vi "Main.vi"(8 "error in":errorcluster, 11 "ArduinoOperator in":refnum<class "ArduinoOperator.lvclass">) -> (0 "error out":errorcluster, 3 "ArduinoOperator out":refnum<class "ArduinoOperator.lvclass">)   [LabVIEW 2022 SP3, in "ArduinoOperator.lvclass"]
doc: "The Queued Message Handler of a Worker."
uses:
  ArduinoOperator.lvclass
  C:/Program Files (x86)/National Instruments/LabVIEW 2022/vi.lib/addons/_Workers/Library/Classes/Worker/Worker.lvclass
  <vilib>/addons/_Workers/Library/Classes/Worker/Worker.lvclass/Worker.ctl
  <vilib>/addons/_Workers/Library/Classes/Message/Priority.ctl
  ArduinoOperator.lvclass/ArduinoOperator.ctl
  <vilib>/MakerHub/LINX/Public/Peripherals/Analog/Analog Read 1 Chan.vi
  <vilib>/MakerHub/LINX/Public/Peripherals/Digital/Digital Read 1 Chan.vi
  <vilib>/MakerHub/LINX/Public/Peripherals/Digital/Digital Write 1 Chan.vi
  <vilib>/MakerHub/LINX/Public/Peripherals/Analog/Analog Read N Chans.vi
  <vilib>/MakerHub/LINX/Public/Peripherals/Digital/Digital Read N Chans.vi
  <vilib>/MakerHub/LINX/Public/Peripherals/Digital/Digital Write N Chans.vi
  <vilib>/MakerHub/LINX/Private/Local IO/LinxAnalogRead.vi
  <vilib>/MakerHub/LINX/Public/Utilities/Check Channel.vi
  <vilib>/MakerHub/LINX/Private/Local IO/LinxDigitalRead.vi
  <vilib>/MakerHub/LINX/Private/Local IO/LinxDigitalWrite.vi
  <vilib>/addons/_Workers/Library/Classes/Message/Enqueue Message to Self v2.vi
  <vilib>/MakerHub/LINX/Public/Utilities/Open Serial.vi
  <vilib>/MakerHub/LINX/Private/Utilties/Generate Error.vi
  <vilib>/addons/_Workers/Library/Classes/Message/Enqueue Message to Self v2 - Array.vi
  Initialization Data.ctl
  <vilib>/addons/_Workers/Library/Classes/Worker/Worker.lvclass
  <vilib>/addons/_Workers/Library/Classes/Message/Message.lvclass
  <vilib>/MakerHub/LINX/LMH-LINX.lvlib
  C:/Program Files (x86)/National Instruments/LabVIEW 2022/vi.lib/addons/_Workers/Library/Classes/Workers Object/Workers Object.lvclass
  C:/Users/chrismadlax/Desktop/LVSampleCode/ArduinoController/Workers/ArduinoOperator/ArduinoOperator.lvclass
  <vilib>/addons/_Workers/Library/Classes/Message Queue/Message Queue.lvclass
panel:
  out "Target":bool
  in  "TimerON":bool
  in  "TimerCount(ms)":i32=1000
  out "Loop Rate (Hz)":u32
  in  "Close":bool
  in  "Link":bool
  in  "AI Channel":u8
  out "Analog Data":dbl(graph)
  in  "DI Channel":u8=2
  out "DI Value":bool
  in  "DO Value":bool
  in  "DO Channel":u8=3
  in  "Serial Port":refnum<visa-resource-name>
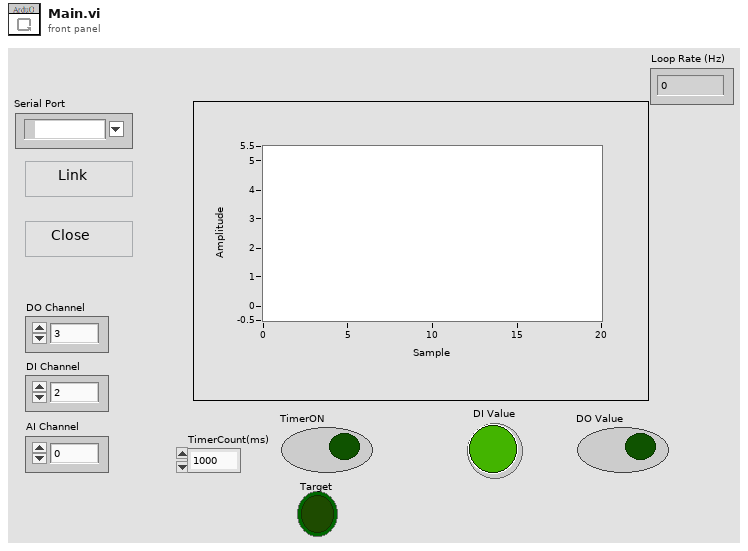
[diagram p1: front panel]
types:
  T1 = typedef "ArduinoOperator.lvclass/Initialization Data.ctl" = cluster{"String":string}
  T2 = typedef "Workers.lvlib/Message.lvclass/Priority.ctl" = enum16{"Low", "Normal", "High"}
  T3 = typedef "Workers.lvlib/Case Label.ctl" = string
  T4 = typedef "LMH-LINX.lvlib/LINX Ref.ctl" = cluster{"IO":T5, "Interface":T6, "LINX Device Config":T7}
  T5 = typedef "LMH-LINX.lvlib/Platform.ctl" = enum16{"Remote", "Local"}
  T6 = typedef "LMH-LINX.lvlib/Interface.ctl" = enum16{"Serial", "TCP"}
  T7 = typedef "LMH-LINX.lvlib/Device.lvlib/LINX Device Config.ctl" = cluster{"Interface":T6, "COM Port":refnum<visa-resource-name>, "TCP Configuration":T8, "Device Family":u8, "Device ID":u8, "Device Name":string, "TCP Ref":refnum<k5>, "Channels":T9}
  T8 = typedef "LMH-LINX.lvlib/Device.lvlib/TCP Config.ctl" = cluster{"IP Address":string, "Port":u16}
  T9 = typedef "LMH-LINX.lvlib/Channels.ctl" = cluster{"DI":u8[], "DO":u8[], "AI":u8[], "AO":u8[], "PWM":u8[], "QE":u8[], "UART":u8[], "I2C 2":u8[], "SPI":u8[], "CAN":u8[], "Servo":u8[], "AI Ref (V)":dbl, "AI Resolution (Bits)":u8, "AO Ref (V)":dbl, "AO Resolution (Bits)":u8}
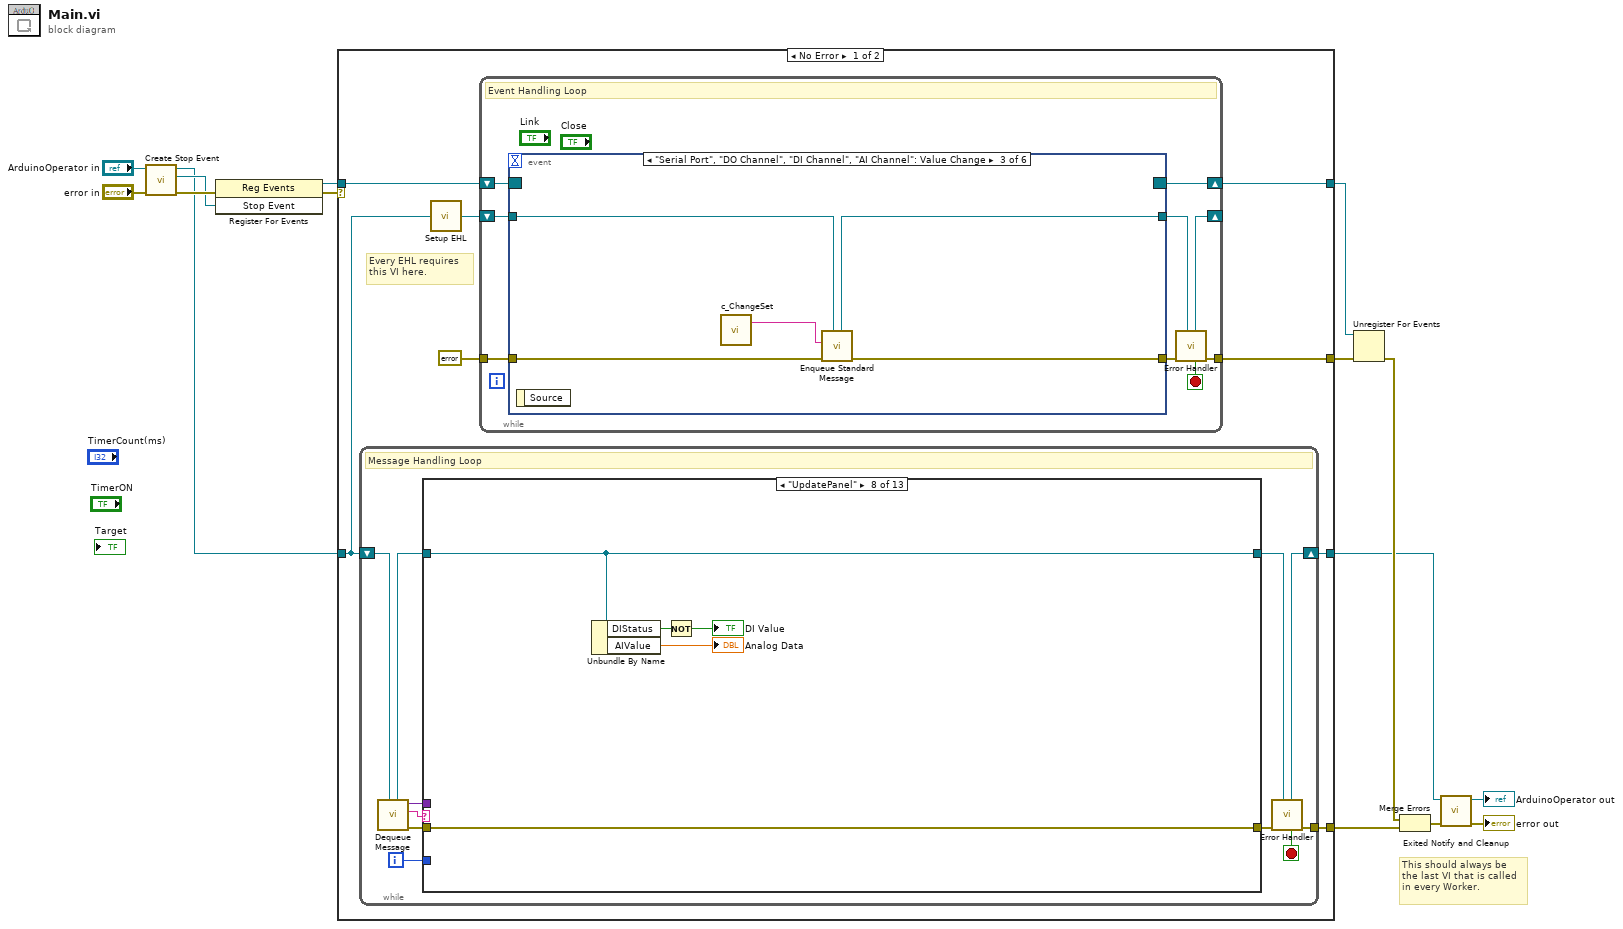
[diagram p0: block diagram]
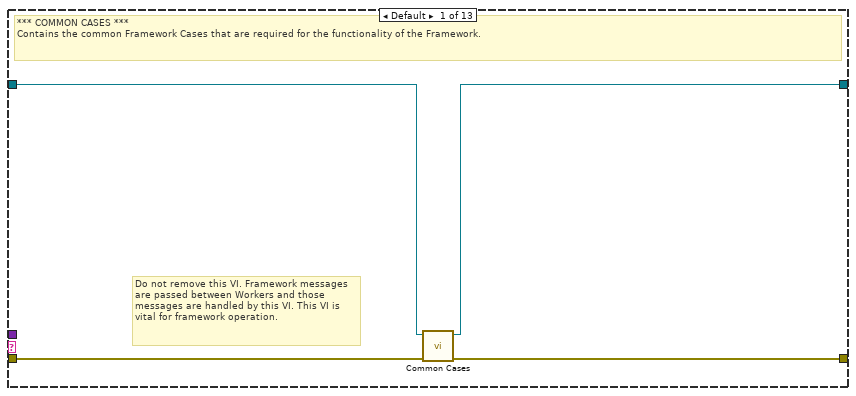
[diagram p2: hidden frame]
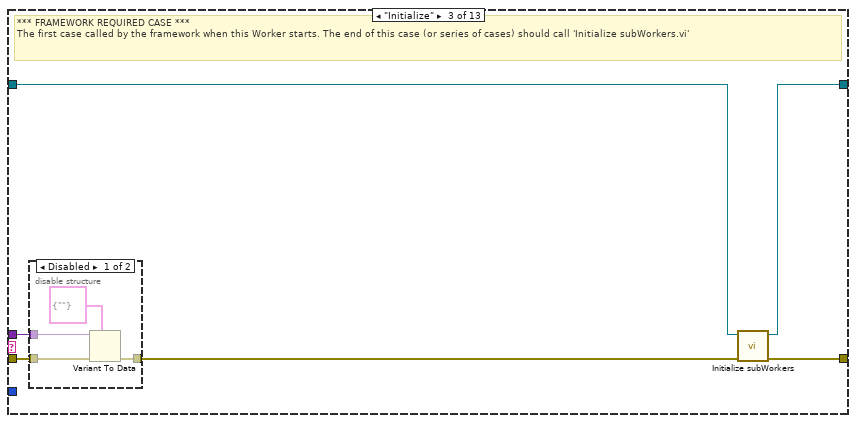
[diagram p4: hidden frame]
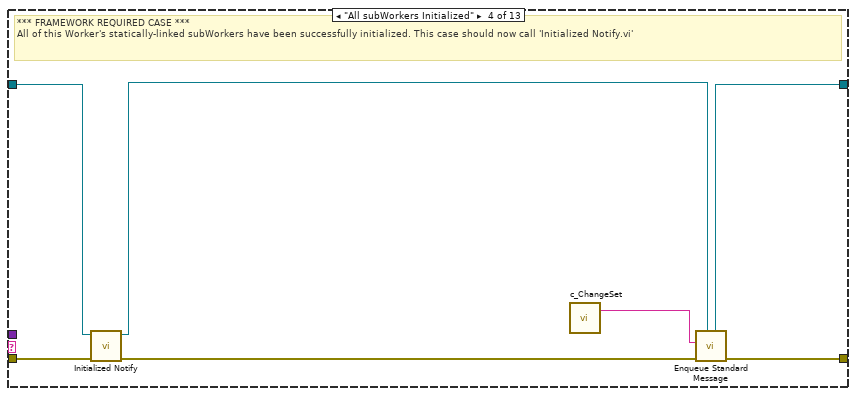
[diagram p6: hidden frame]
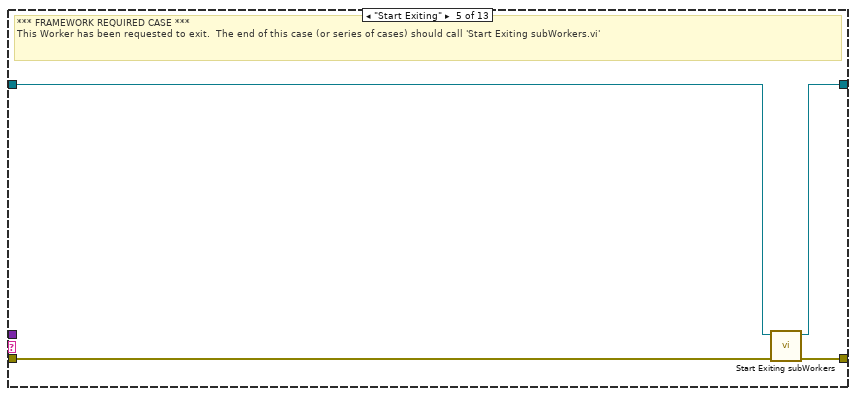
[diagram p7: hidden frame]
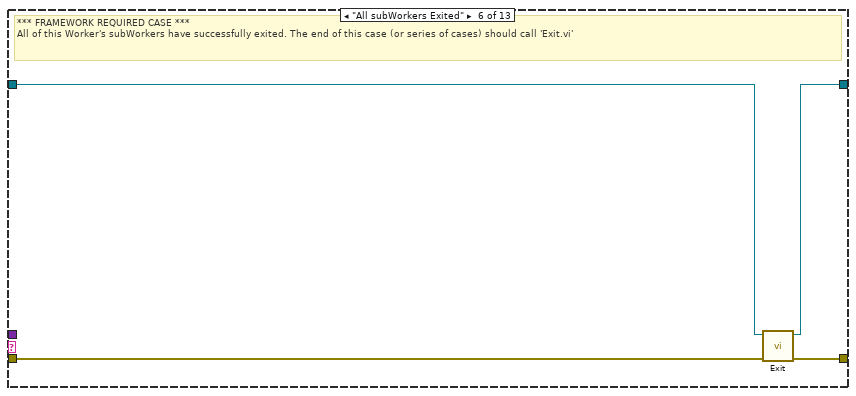
[diagram p8: hidden frame]
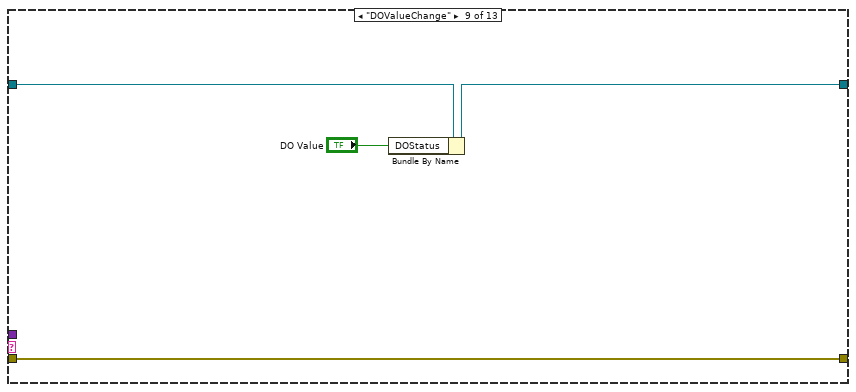
[diagram p10: hidden frame]
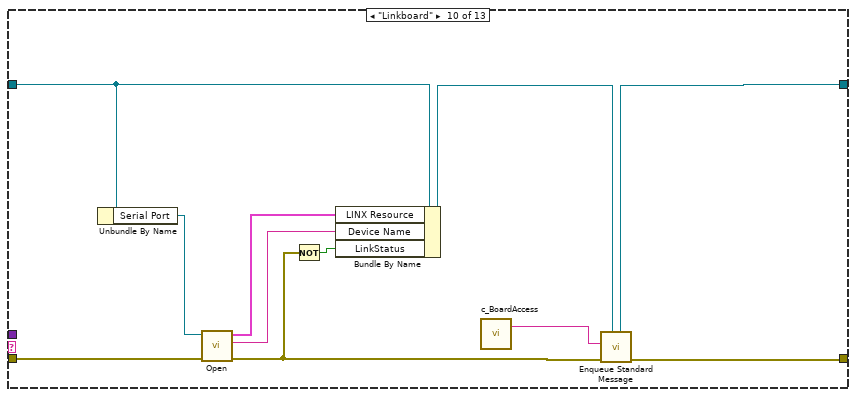
[diagram p11: hidden frame]
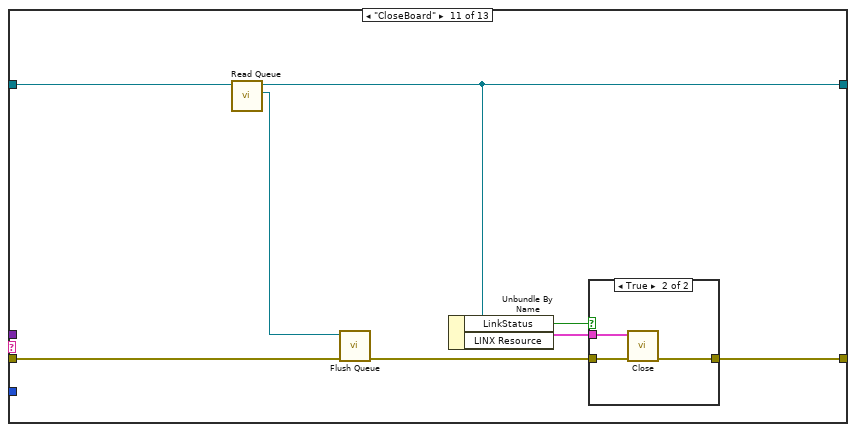
[diagram p12: hidden frame]
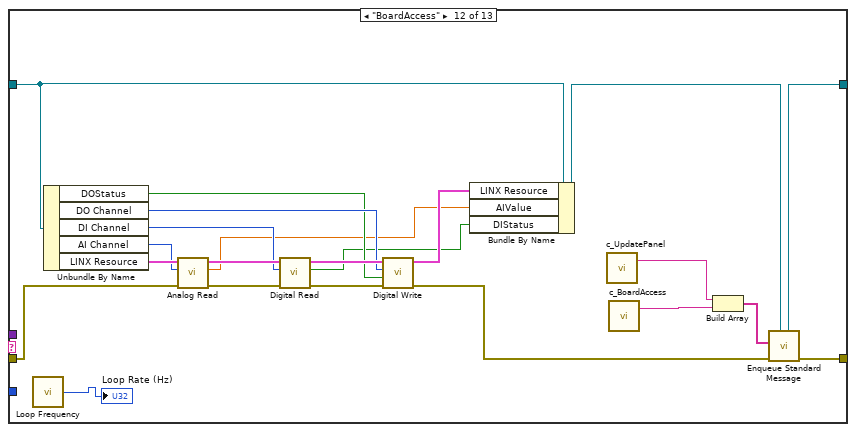
[diagram p14: hidden frame]
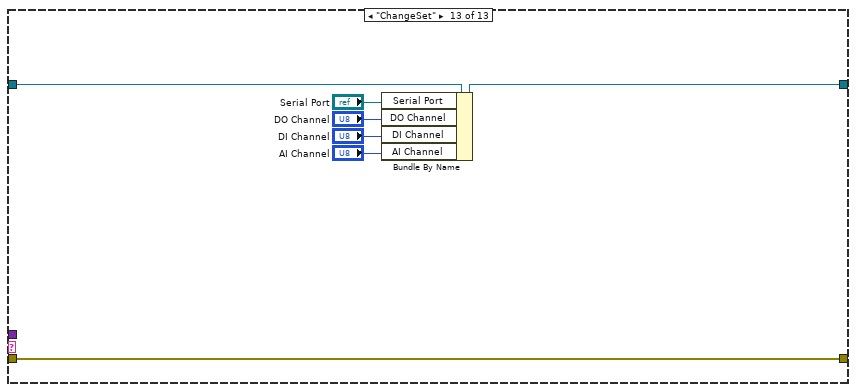
[diagram p15: hidden frame]
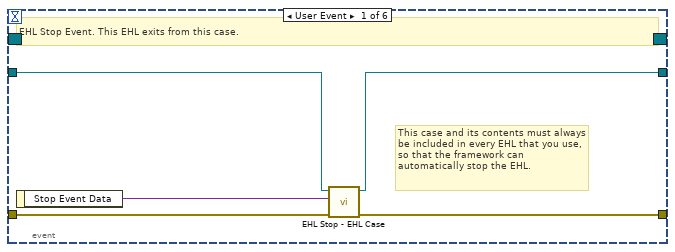
[diagram p16: hidden frame]
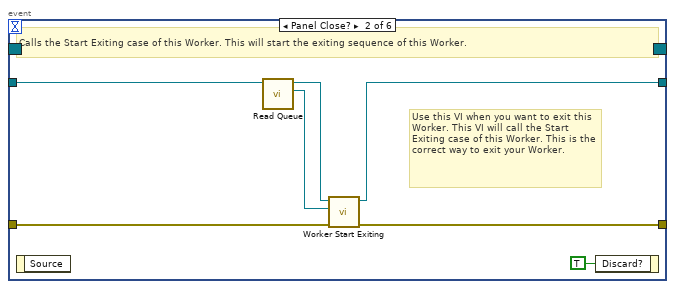
[diagram p17: hidden frame]
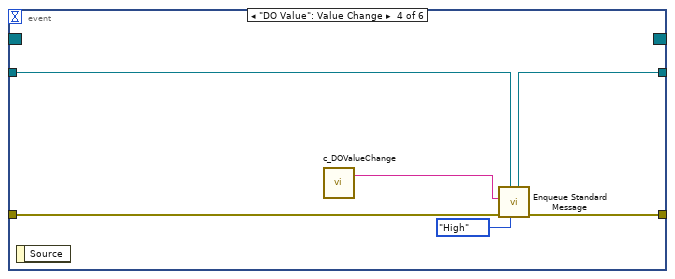
[diagram p18: hidden frame]
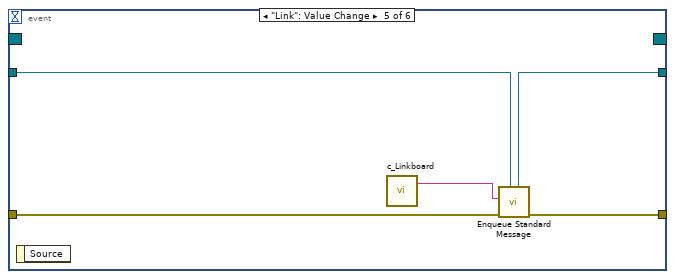
[diagram p19: hidden frame]
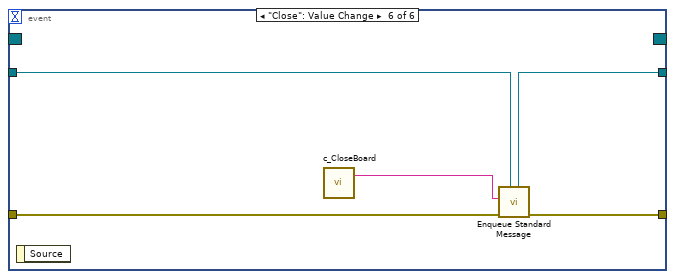
[diagram p20: hidden frame]
diagram:
  # "This should always be the last VI that is called in every Worker."
  n1 = call-dynamic "Create Stop Event.vi"("error in"="error in", "Worker"="ArduinoOperator in") -> ("error out"=w10:errorcluster, "Stop Event"=w7:refnum<user-event>, "Worker out"=w4:refnum<class "ArduinoOperator.lvclass">)  [unwired: 7 in]
  n2 = register-events(error in=w10, w7) -> (reference out=w9:refnum<event-registration>, error out=w1:errorcluster)  [unwired: 1 in]
  n3 = case shown="No Error" w1 {
    tunnel: w4 -> [w18 w173]
    tunnel: [w16 w174] -> w8
    tunnel: w9 -> [w23 w175]
    tunnel: [w20 w176] -> w14
    tunnel: [w22 w175] -> w13
    tunnel: [w17 w172] -> w11
    selector: w1 -> [_ w176]
    frame No Error {
      # "Every EHL requires\nthis VI here."
      n4 = while {
        shift-right: [w32] -> w17
        shift-left: w18 -> [w34]
        tunnel: [w33] -> w16
        i -> [w24]
        stop <- w25 stop-if-true
        # "Message Handling Loop"
        n5 = call-dynamic "Dequeue Message.vi"("Worker"=w34) -> ("error out"=w31:errorcluster, "Case out"=w26:string, "Data out"=w27:variant, "Worker out"=w29:refnum<class "ArduinoOperator.lvclass">)  [unwired: 6 in, 1 out]
        n6 = case "Worker MHL Case Structure (DO NOT CHANGE LABEL NAME)" shown="\"UpdatePanel\"" w26 {
          tunnel: w31 -> [w38 w39 w44 w57 w59 w66 w67 w73 w77 w88 w92 w115 w129]
          tunnel: [w37 w39 w46 w55 w62 w65 w67 w73 w77 w80 w93 w105 w129] -> w30
          tunnel: w29 -> [w36 w40 w43 w58 w60 w64 w68 w72 w76 w87 w96 w119 w128]
          tunnel: [w35 w40 w45 w53 w61 w63 w68 w72 w75 w81 w90 w107 w127] -> w28
          tunnel: w27 -> [_ _ w41 _ _ _ _ _ _ _ _ _ _]
          tunnel: w24 -> [_ _ _ _ _ _ _ _ _ _ _ _ _]
          frame Default {
            # "Do not remove this VI. Framework messages are passed between Workers and those messages are handled by this VI. This VI is vital for framework operation."
            # "*** COMMON CASES ***\nContains the common Framework Cases that are required for the functionality of the Framework."
            n7 = call-dynamic "Common Cases.vi"("error in"=w38, "Worker in"=w36) -> ("error out"=w37:errorcluster, "Worker out"=w35:refnum<class "ArduinoOperator.lvclass">)  [unwired: 8 in]
          }
          frame "------ FRAMEWORK REQUIRED CASES ------" {
            # "Start of Framework Required Cases"
          }
          frame "Initialize" {
            # "*** FRAMEWORK REQUIRED CASE ***\nThe first case called by the framework when this Worker starts. The end of this case (or series of cases) should call 'Initialize subWorkers.vi'"
            n8 = disable-structure shown="Disabled" {
              disable-tunnel: w44 -> [w50 w51]
              disable-tunnel: [w49 w51] -> w42
              disable-tunnel: w41 -> [w48 _]
              frame Disabled {
                n9 = Variant To Data(error in=w50, type=T1 {"String"=""} ("Initialization Data"), Variant=w48) -> (error out=w49:errorcluster)  [unwired: 1 out]
              }
              frame Enabled {
              }
            }
            n10 = call-dynamic "Initialize subWorkers.vi"("error in"=w42, "Worker"=w43) -> ("error out"=w46:errorcluster, "dup Worker out"=w45:refnum<class "ArduinoOperator.lvclass">)  [unwired: 8 in]
          }
          frame "All subWorkers Initialized" {
            # "*** FRAMEWORK REQUIRED CASE ***\nAll of this Worker's statically-linked subWorkers have been successfully initialized. This case should now call 'Initialized Notify.vi'"
            n11 = call-dynamic "Initialized Notify.vi"("error in"=w57, "Worker"=w58) -> ("error out"=w56:errorcluster, "dup Worker out"=w54:refnum<class "ArduinoOperator.lvclass">)  [unwired: 8 in]
            n12 = call "c_ChangeSet.vi"() -> ("Case Label"=w52:T3)  [unwired: 1 in]
            n13 = call-poly <vilib>:"Enqueue Standard Message.vi"("Worker"=w54, "error in"=w56, "Case Label"=w52) -> ("error out"=w55:errorcluster, "dup Worker out"=w53:refnum<class "ArduinoOperator.lvclass">)  [unwired: 7 in]
          }
          frame "Start Exiting" {
            # "*** FRAMEWORK REQUIRED CASE ***\nThis Worker has been requested to exit.  The end of this case (or series of cases) should call 'Start Exiting subWorkers.vi'"
            n14 = call-dynamic "Start Exiting subWorkers.vi"("error_in"=w59, "Worker"=w60) -> ("error out"=w62:errorcluster, "dup Worker out"=w61:refnum<class "ArduinoOperator.lvclass">)  [unwired: 8 in]
          }
          frame "All subWorkers Exited" {
            # "*** FRAMEWORK REQUIRED CASE ***\nAll of this Worker's subWorkers have successfully exited. The end of this case (or series of cases) should call 'Exit.vi'"
            n15 = call-dynamic "Exit.vi"("error_in"=w66, "Worker"=w64) -> ("error out"=w65:errorcluster, "dup Worker out"=w63:refnum<class "ArduinoOperator.lvclass">)  [unwired: 8 in]
          }
          frame "-----------------------------------------------" {
            # "End of Framework Required Cases"
          }
          frame "UpdatePanel" {
            n16 = Unbundle By Name(w72) -> ("DIStatus"=w71:bool, "AIValue"=→"Analog Data":dbl)
            n17 = Not(x=w71) -> (.not. x?=→"DI Value":bool)
          }
          frame "DOValueChange" {
            n18 = Bundle By Name(cluster=w76, "DOStatus"="DO Value") -> (w75:refnum<class "ArduinoOperator.lvclass">)
          }
          frame "Linkboard" {
            n19 = Unbundle By Name(w87) -> ("Serial Port"=w86:refnum<visa-resource-name>)
            n20 = call-poly <vilib>:"Open.vi"("Error In"=w88, "Serial Port"=w86) -> ("Error Out"=w79:errorcluster, "Device Name"=w83:string, "LINX Resource"=w84:T4)  [unwired: 7 in]
            n21 = Not(x=w79) -> (.not. x?=w82:bool)
            n22 = Bundle By Name(cluster=w87, "LINX Resource"=w84, "Device Name"=w83, "LinkStatus"=w82) -> (w85:refnum<class "ArduinoOperator.lvclass">)
            n23 = call "c_BoardAccess.vi"() -> ("Case Label"=w78:T3)  [unwired: 1 in]
            n24 = call-poly <vilib>:"Enqueue Standard Message.vi"("Worker"=w85, "error in"=w79, "Case Label"=w78) -> ("error out"=w80:errorcluster, "dup Worker out"=w81:refnum<class "ArduinoOperator.lvclass">)  [unwired: 7 in]
          }
          frame "CloseBoard" {
            n25 = call <vilib>:"Read Queue.vi"("Worker"=w96) -> ("Message Queue out"=w89:refnum<class "Message Queue.lvclass">, "dup Worker out"=w90:refnum<class "ArduinoOperator.lvclass">)  [unwired: 9 in]
            n26 = call <vilib>:"Flush Queue.vi"("error in (no error)"=w92, "Message Queue"=w89) -> ("error out"=w91:errorcluster)  [unwired: 7 in, 2 out]
            n27 = Unbundle By Name(w90) -> ("LinkStatus"=w94:bool, "LINX Resource"=w95:T4)
            n28 = case shown="True" w94 {
              tunnel: w95 -> [_ w100]
              tunnel: w91 -> [w97 w99]
              tunnel: [w97 w98] -> w93
              frame False {
              }
              frame True {
                n29 = call <vilib>:"Close.vi"("Error In"=w99, "LINX Resource"=w100) -> ("Error Out"=w98:errorcluster)  [unwired: 9 in]
              }
            }
          }
          frame "BoardAccess" {
            n30 = call <vilib>:"Loop Frequency.vi"() -> ("Loop Rate (Hz)"=→"Loop Rate (Hz)":u32)
            n31 = Unbundle By Name(w119) -> ("DOStatus"=w112:bool, "DO Channel"=w113:u8, "DI Channel"=w114:u8, "AI Channel"=w118:u8, "LINX Resource"=w120:T4)
            n32 = call-poly <vilib>:"Analog Read.vi"("Error In"=w115, "Analog Channel"=w118, "LINX Resource"=w120) -> ("Error Out"=w122:errorcluster, "Voltage"=w109:dbl, "LINX Resource"=w117:T4)  [unwired: 5 in, 1 out]
            n33 = call-poly <vilib>:"Digital Read.vi"("Error In"=w122, "DI Channel"=w114, "LINX Resource"=w117) -> ("Error Out"=w121:errorcluster, "DI Value"=w108:bool, "LINX Resource"=w116:T4)  [unwired: 6 in]
            n34 = call-poly <vilib>:"Digital Write.vi"("Error In"=w121, "Output Value"=w112, "DO Channel"=w113, "LINX Resource"=w116) -> ("Error Out"=w106:errorcluster, "LINX Resource"=w110:T4)  [unwired: 6 in]
            n35 = Bundle By Name(cluster=w119, "LINX Resource"=w110, "AIValue"=w109, "DIStatus"=w108) -> (w111:refnum<class "ArduinoOperator.lvclass">)
            n36 = call "c_UpdatePanel.vi"() -> ("Case Label"=w103:T3)  [unwired: 1 in]
            n37 = call "c_BoardAccess.vi"() -> ("Case Label"=w102:T3)  [unwired: 1 in]
            n38 = Build Array(w103, w102) -> (w101:T3[])
            n39 = call-poly <vilib>:"Enqueue Standard Message.vi"("Worker"=w111, "error in"=w106, "Case Label []"=w101) -> ("error out"=w105:errorcluster, "dup Worker out"=w107:refnum<class "ArduinoOperator.lvclass">)  [unwired: 7 in]
          }
          frame "ChangeSet" {
            n40 = Bundle By Name(cluster=w128, "Serial Port"="Serial Port", "DO Channel"="DO Channel", "DI Channel"="DI Channel", "AI Channel"="AI Channel") -> (w127:refnum<class "ArduinoOperator.lvclass">)
          }
        }
        n41 = call-dynamic "Error Handler.vi"("Worker"=w28, "error_in"=w30) -> ("error out"=w33:errorcluster, "Stop Loop"=w25:bool, "Worker out"=w32:refnum<class "ArduinoOperator.lvclass">)  [unwired: 7 in]
      }
      n42 = call-dynamic "Setup EHL.vi"("Worker"=w18) -> ("Worker out"=w19:refnum<class "ArduinoOperator.lvclass">)  [unwired: 14 in]
      n43 = while "Event Handling Loop" {
        shift-right: [w138] -> w22
        shift-left: w23 -> [w137]
        tunnel: [w133] -> w20
        tunnel: errorcluster {"status"=FALSE, "code"=0, "source"=""} ("error constant") -> [w135]
        shift-right: [w131] -> _
        shift-left: w19 -> [w136]
        stop <- w130 stop-if-true
        # "Event Handling Loop"
        n44 = event shown="[2] \"Serial Port\", \"DO Channel\", \"DI Channel\", \"AI Channel\": Value Change" {
          selector: w137 -> [_ _ _ _ _ _]
          dyn-events: [_ _ _ _ _ _] -> w138
          timeout: _ -> [_ _ _ _ _ _]
          tunnel: [w142 w149 w154 w160 w165 w170] -> w134
          tunnel: w135 -> [w143 w148 w155 w161 w166 w171]
          tunnel: w136 -> [w141 w147 w153 w159 w164 w169]
          tunnel: [w140 w146 w152 w158 w163 w168] -> w132
          event User Event {
            # "This case and its contents must always be included in every EHL that you use, so that the framework can automatically stop the EHL."
            # "EHL Stop Event. This EHL exits from this case."
            n45 = event-data() -> ("Stop Event Data"=w139:variant)  [unwired: 1 in]
            n46 = call <vilib>:"EHL Stop - EHL Case.vi"("error in"=w143, "Stop Event Data"=w139, "Worker"=w141) -> ("error out"=w142:errorcluster, "Worker out"=w140:refnum<class "ArduinoOperator.lvclass">)  [unwired: 7 in]
          }
          event Panel Close? {
            # "Use this VI when you want to exit this Worker. This VI will call the Start Exiting case of this Worker. This is the correct way to exit your Worker."
            # "Calls the Start Exiting case of this Worker. This will start the exiting sequence of this Worker."
            n47 = event-data() -> ()  [unwired: 1 in, 1 out]
            n48 = call <vilib>:"Read Queue.vi"("Worker"=w147) -> ("Message Queue out"=w144:refnum<class "Message Queue.lvclass">, "dup Worker out"=w145:refnum<class "ArduinoOperator.lvclass">)  [unwired: 9 in]
            n49 = call-dynamic "Worker Start Exiting.vi"("error_in"=w148, "Message Queue"=w144, "Worker"=w145) -> ("error out"=w149:errorcluster, "dup Worker out"=w146:refnum<class "ArduinoOperator.lvclass">)  [unwired: 7 in]
            n50 = event-data("Discard?"=TRUE) -> ()  [unwired: 1 in, 1 out]
          }
          event "Serial Port", "DO Channel", "DI Channel", "AI Channel": Value Change {
            n51 = event-data() -> ()  [unwired: 1 in, 1 out]
            n52 = call "c_ChangeSet.vi"() -> ("Case Label"=w151:T3)  [unwired: 1 in]
            n53 = call-poly <vilib>:"Enqueue Standard Message.vi"("Worker"=w153, "error in"=w155, "Case Label"=w151) -> ("error out"=w154:errorcluster, "dup Worker out"=w152:refnum<class "ArduinoOperator.lvclass">)  [unwired: 7 in]
          }
          event "DO Value": Value Change {
            n54 = event-data() -> ()  [unwired: 1 in, 1 out]
            n55 = call "c_DOValueChange.vi"() -> ("Case Label"=w157:T3)  [unwired: 1 in]
            n56 = call-poly <vilib>:"Enqueue Standard Message.vi"("Priority (Normal)"=Priority."High", "Worker"=w159, "error in"=w161, "Case Label"=w157) -> ("error out"=w160:errorcluster, "dup Worker out"=w158:refnum<class "ArduinoOperator.lvclass">)  [unwired: 6 in]
          }
          event "Link": Value Change {
            n57 = event-data() -> ()  [unwired: 1 in, 1 out]
            n58 = call "c_Linkboard.vi"() -> ("Case Label"=w162:T3)  [unwired: 1 in]
            n59 = call-poly <vilib>:"Enqueue Standard Message.vi"("Worker"=w164, "error in"=w166, "Case Label"=w162) -> ("error out"=w165:errorcluster, "dup Worker out"=w163:refnum<class "ArduinoOperator.lvclass">)  [unwired: 7 in]
          }
          event "Close": Value Change {
            n60 = event-data() -> ()  [unwired: 1 in, 1 out]
            n61 = call "c_CloseBoard.vi"() -> ("Case Label"=w167:T3)  [unwired: 1 in]
            n62 = call-poly <vilib>:"Enqueue Standard Message.vi"("Worker"=w169, "error in"=w171, "Case Label"=w167) -> ("error out"=w170:errorcluster, "dup Worker out"=w168:refnum<class "ArduinoOperator.lvclass">)  [unwired: 7 in]
          }
        }
        n63 = call-dynamic "Error Handler.vi"("Worker"=w132, "error_in"=w134) -> ("error out"=w133:errorcluster, "Stop Loop"=w130:bool, "Worker out"=w131:refnum<class "ArduinoOperator.lvclass">)  [unwired: 7 in]
      }
    }
    frame Error {
      n64 = call-dynamic "Error Handler.vi"("Worker"=w173, "error_in"=w176) -> ("error out"=w174:errorcluster, "Worker out"=w172:refnum<class "ArduinoOperator.lvclass">)  [unwired: 7 in, 1 out]
    }
  }
  n65 = Unregister For Events(event registration refnum=w13, error in=w14) -> (error out=w15:errorcluster)
  n66 = Merge Errors(w15, w8) -> (w12:errorcluster)
  n67 = call-dynamic "Exited Notify and Cleanup.vi"("error_in"=w12, "Worker"=w11) -> ("error out"=→"error out":errorcluster, "dup Worker out"=→"ArduinoOperator out":refnum<class "ArduinoOperator.lvclass">)  [unwired: 8 in]
